vi "runtest add timing.vi"(8 "error in (no error)":errorcluster, 9 "Start Tick, ms (0)":u32, 10 "Function (\"\")":string, 11 "POST (empty)":T1) -> (0 "error out":errorcluster, 3 "POST out":T1)   [LabVIEW 2011]
uses:
  Addons/internet/utils/keyedarr.llb/Keyed Array.ctl
  Addons/internet/utils/strutil.llb/Case Matching.ctl
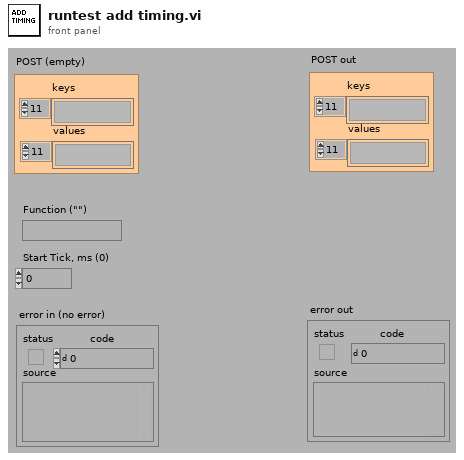
[diagram p1: front panel]
types:
  T1 = typedef "Keyed Array.ctl" = cluster{"keys":string[], "values":string[]}
  T2 = typedef "Case Matching.ctl" = enum16{"a != A", "a == A", "system"}
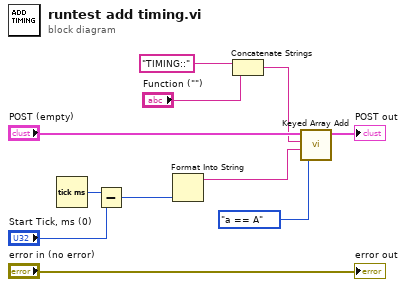
[diagram p0: block diagram]
diagram:
  n1 = Tick Count (ms)() -> (millisecond timer value=w8:u32)
  n2 = Subtract(x=w8, y="Start Tick, ms (0)") -> (x-y=w6:u32)
  n3 = Format Into String(w6) -> (resulting string=w1:string)  [unwired: 3 in, 1 out]
  n4 = Concatenate Strings("TIMING::", "Function (\"\")") -> (w2:string)
  n5 = call "Keyed Array Add.vi"("case matching (sensitive)"=Case_Matching."a == A", "value"=w1, "key"=w2, "array in"="POST (empty)") -> ("array out"=→"POST out":T1)  [unwired: 3 out]
  "error out" <- "error in (no error)"
